vi "publishGrating.vi"(8 "error in (no error)":errorcluster, 10 "GratingType":T1, 11 "Monochromator in":refnum<class "Monochromator.lvclass">) -> (0 "error out":errorcluster, 3 "Monochromator out":refnum<class "Monochromator.lvclass">)   [LabVIEW 2016, in "Monochromator.lvclass"]
uses:
  Monochromator.lvclass
  Typedefs/GratingType.ctl
  Monochromator.lvclass/Monochromator.ctl
  MonoPubSubData/MonoPubSubData.lvclass/MonoPubSubData.ctl
  MonoPubSubData/MonoPubSubData.lvclass
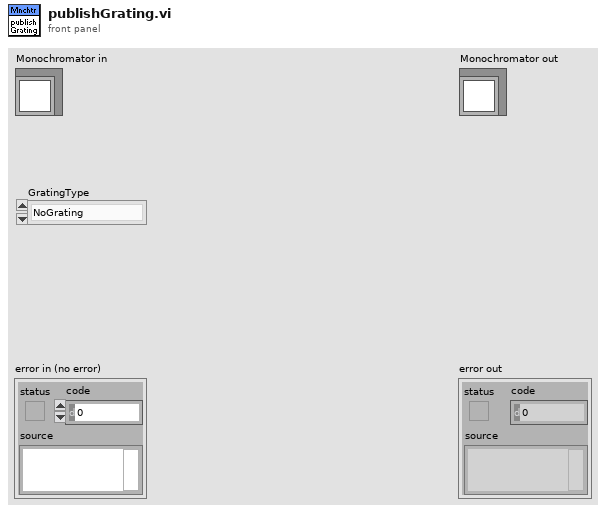
[diagram p1: front panel]
types:
  T1 = typedef "GratingType.ctl" = enum16{"NoGrating", "Red", "Blue", "Mirror"}
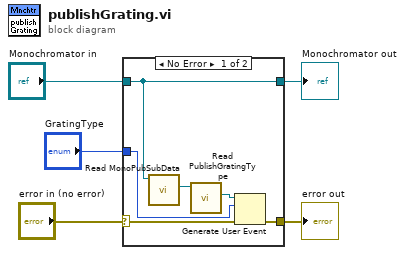
[diagram p0: block diagram]
diagram:
  n1 = case shown="No Error" "error in (no error)" {
    selector: "error in (no error)" -> [w7 w13]
    tunnel: [w6 w13] -> w4
    tunnel: [w11 w12] -> w2
    tunnel: "Monochromator in" -> [w11 w12]
    tunnel: "GratingType" -> [w8 _]
    frame No Error {
      n2 = call "Read MonoPubSubData.vi"("Monochromator in"=w11) -> ("MonoPubSubData.lvclass"=w10:refnum<class "MonoPubSubData.lvclass">)  [unwired: 8 in, 2 out]
      n3 = call "Read PublishGratingType.vi"("MonoPubSubData in"=w10) -> ("PublishGratingType"=w9:refnum<user-event>)  [unwired: 8 in, 2 out]
      n4 = Generate User Event(user event=w9, event data cluster=w8, error in=w7) -> (error out=w6:errorcluster)  [unwired: 1 in, 1 out]
    }
    frame Error {
    }
  }
  "error out" <- w4
  "Monochromator out" <- w2
